vi "g_Panel Qarr.vi"(9 "VI Address":u16, 10 "Console Q":refnum<queue>, 11 "Operation":T1(ring)=enum."Get") -> (2 "Console Q out":refnum<queue>)   [LabVIEW 2015, in "EditPanel API.lvlib" / "EditPanel API.lvclass"]
uses:
  EditPanel_class/EditPanel API.lvclass
  Console_Q Data Type.ctl
  Console Reply/Console Reply/Console Reply.lvclass
  Panel Control_Interface/Panel_interface/Panel Controller Interface.lvclass
  Console.lvclass
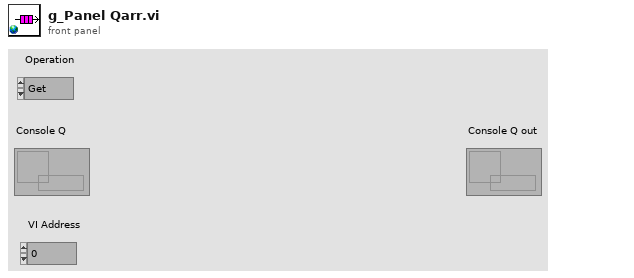
[diagram p1: front panel]
types:
  T1 = enum16{"Attach", "Detach", "Flush", "Update", "Get"}
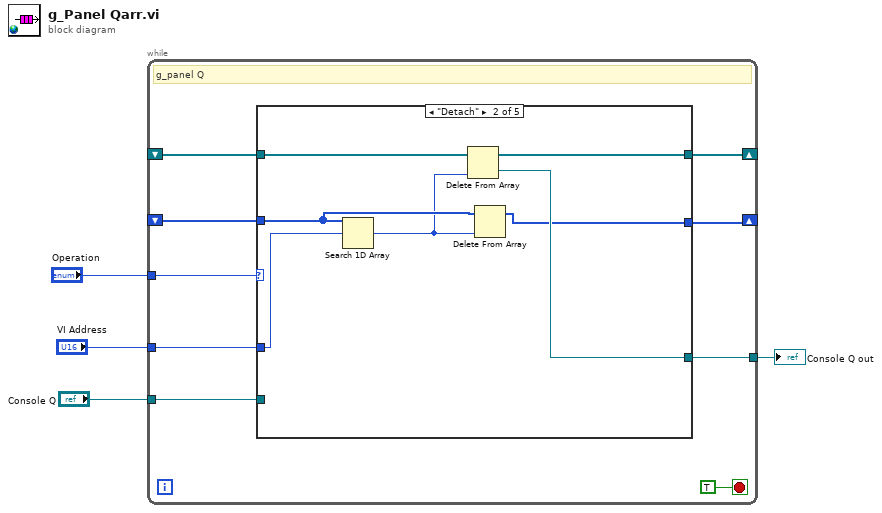
[diagram p0: block diagram]
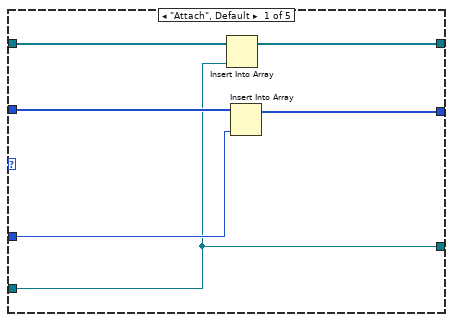
[diagram p2: hidden frame]
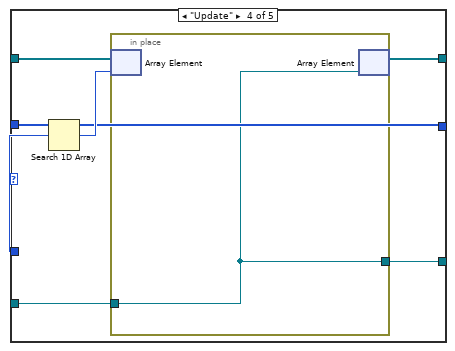
[diagram p4: hidden frame]
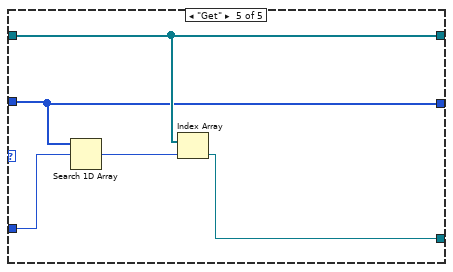
[diagram p5: hidden frame]
diagram:
  n1 = while {
    shift-right: [w6] -> _
    shift-left: _ -> [w11]
    tunnel: "Operation" -> [w12]
    tunnel: "VI Address" -> [w9]
    tunnel: "Console Q" -> [w8]
    shift-right: [w7] -> _
    shift-left: _ -> [w10]
    tunnel: [w5] -> w1
    stop <- TRUE stop-if-true
    # "g_panel Q"
    n2 = case shown="\"Detach\"" w12 {
      tunnel: w11 -> [w19 w25 _ w33 w36]
      tunnel: w10 -> [w18 w22 _ w28 w35]
      tunnel: w9 -> [w17 w26 _ w32 w39]
      tunnel: w8 -> [w14 _ _ w30 _]
      tunnel: [w16 w20 _ w28 w35] -> w7
      tunnel: [w15 w24 _ w29 w36] -> w6
      tunnel: [w14 w23 _ w27 w37] -> w5
      frame "Attach", Default {
        n3 = Insert Into Array(array=w19, new element=w14) -> (w15:refnum<queue>[])  [unwired: 1 in]
        n4 = Insert Into Array(array=w18, new element=w17) -> (w16:u16[])  [unwired: 1 in]
      }
      frame "Detach" {
        n5 = Search 1D Array(1D array=w22, element=w26) -> (index of element=w21:i32)  [unwired: 1 in]
        n6 = Delete From Array(array=w25, index=w21) -> (deleted portion=w23:refnum<queue>, array with subset deleted=w24:refnum<queue>[])  [unwired: 1 in]
        n7 = Delete From Array(array=w22, index=w21) -> (array with subset deleted=w20:u16[])  [unwired: 1 in, 1 out]
      }
      frame "Flush" {
      }
      frame "Update" {
        n8 = Search 1D Array(1D array=w28, element=w32) -> (index of element=w31:i32)  [unwired: 1 in]
        n9 = in-place {
          in-place-border: w30 -> [w34]
          in-place-border: [w34] -> w27
          n10 = in-place-array #1(w33, w31) -> ()  [unwired: 1 out]
          n11 = in-place-array #1(w34) -> (w29:refnum<queue>[])  [unwired: 1 out]
        }
      }
      frame "Get" {
        n12 = Search 1D Array(1D array=w35, element=w39) -> (index of element=w38:i32)  [unwired: 1 in]
        n13 = Index Array(array=w36, index=w38) -> (element=w37:refnum<queue>)
      }
    }
  }
  "Console Q out" <- w1
